vi "CleanUp.vi"(8 "error in (no error)":errorcluster, 11 "Prueba02 in":refnum<class "Prueba02.lvclass">) -> (0 "error out":errorcluster, 3 "Prueba02 out":refnum<class "Prueba02.lvclass">)   [LabVIEW 2019, in "Prueba02.lvclass"]
uses:
  Prueba02.lvclass
  C:/Users/ivan_/Documents/procal/Pruebas/Prueba/Prueba.lvclass
  Prueba/Prueba.lvclass/Prueba.ctl
  Prueba02.lvclass/Prueba02.ctl
  Base de Datos/SQLiteConnector/SQLiteConnection.lvclass
  Base de Datos/Base de Datos.lvclass
  Prueba/Prueba.lvclass
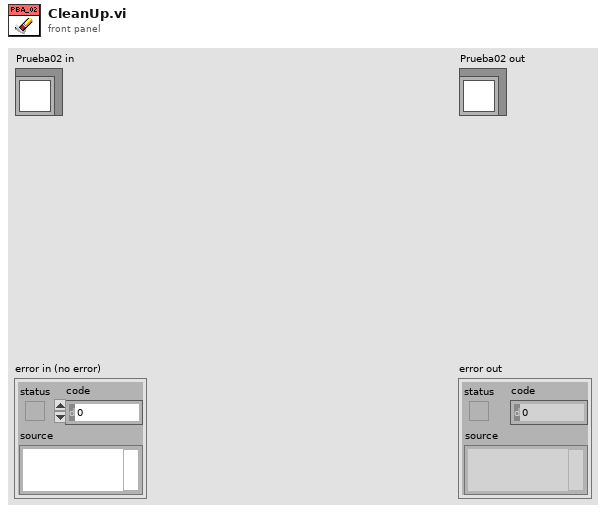
[diagram p1: front panel]
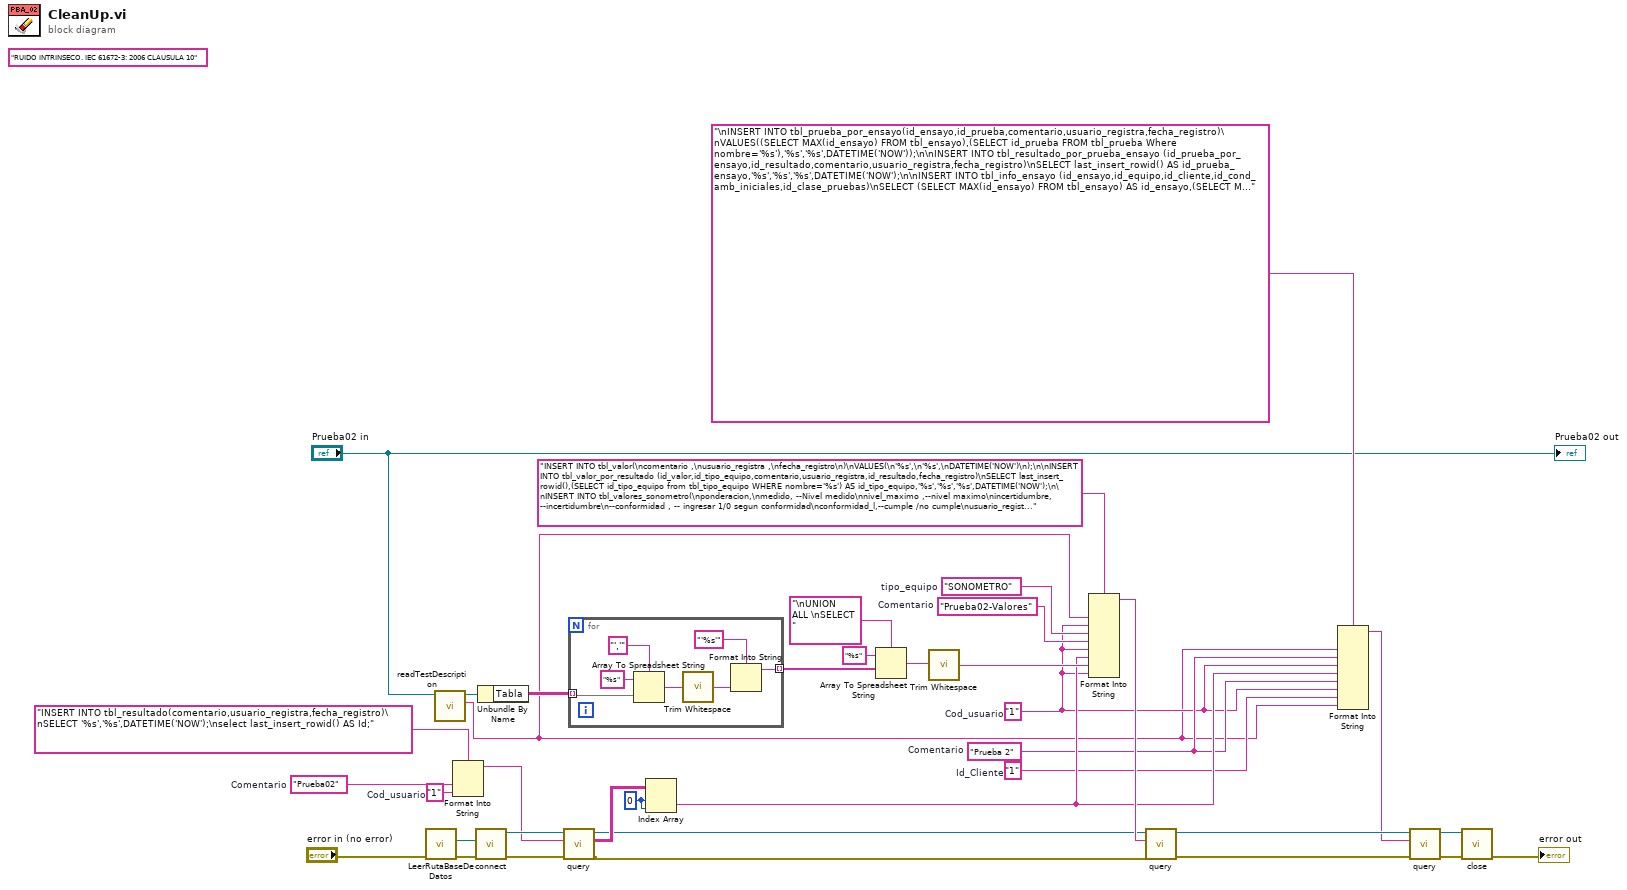
[diagram p0: block diagram]
diagram:
  (unwired) "RUIDO INTRINSECO. IEC 61672-3: 2006 CLAUSULA 10" ("input 2")
  w5 = "1"  # Id_Cliente
  w6 = "Prueba 2"  # Comentario
  w15 = "SONOMETRO"  # tipo_equipo
  w14 = "Prueba02-Valores"  # Comentario
  w21 = 0 ("index (row)")
  w23 = "1"  # Cod_usuario
  w24 = "Prueba02"  # Comentario
  w4 = "1"  # Cod_usuario
  n1 = call "LeerRutaBaseDeDatos.vi"("error in (no error)"="error in (no error)") -> ("error out"=w31:errorcluster, "Database Path"=w30:path)  [unwired: 9 in]
  n2 = call "readTestDescription.vi"("Prueba in"="Prueba02 in") -> ("Test Description"=w1:string, "Prueba out"=w2:refnum<class "Prueba02.lvclass">)  [unwired: 8 in, 1 out]
  n3 = Format Into String(format string="INSERT INTO tbl_resultado(comentario,usuario_registra,fecha_registro)\nSELECT '%s','%s',DATETIME('NOW');\nselect last_insert_rowid() AS Id;" ("SQL Statement"), w24, w23) -> (resulting string=w22:string)  [unwired: 2 in, 1 out]
  n4 = call "connect.vi"("error in (no error)"=w31, "Database Path"=w30) -> ("error out"=w20:errorcluster, "object out"=w26:refnum<class "SQLiteConnection.lvclass">)  [unwired: 8 in]
  n5 = Unbundle By Name(w2) -> ("Tabla"=w32:string[][])
  n6 = call "query.vi"("error in (no error)"=w20, "SQL Statement"=w22, "object in"=w26) -> ("error out"=w17:errorcluster, "result"=w19:string[][], "object out"=w18:refnum<class "SQLiteConnection.lvclass">)  [unwired: 5 in, 1 out]
  n7 = for {
    tunnel: w32 -> [w44] mode=indexing
    tunnel: [w40] -> w35 mode=indexing
    n8 = Array To Spreadsheet String(delimiter (Tab)="','", array=w44, 3:"%s" ("format string")) -> (spreadsheet string=w39:string)
    n9 = call <vilib>:"Trim Whitespace.vi"("string"=w39) -> ("trimmed string"=w38:string)  [unwired: 1 in]
    n10 = Format Into String(format string="'%s'", w38) -> (resulting string=w40:string)  [unwired: 2 in, 1 out]
  }
  n11 = Index Array(array=w19, index (row)=w21, index (col)=w21) -> (element=w7:string)
  n12 = Array To Spreadsheet String(delimiter (Tab)="\nUNION ALL \nSELECT ", array=w35, 3:"%s" ("format string")) -> (spreadsheet string=w34:string)
  n13 = call <vilib>:"Trim Whitespace.vi"("string"=w34) -> ("trimmed string"=w16:string)  [unwired: 1 in]
  n14 = Format Into String(format string="INSERT INTO tbl_valor(\ncomentario ,\nusuario_registra ,\nfecha_registro\n)\nVALUES(\n'%s',\n'%s',\nDATETIME('NOW')\n);\n\nINSERT INTO tbl_valor_por_resultado (id_valor,id_tipo_equipo,comentario,usuario_registra,id_resultado,fecha_registro)\nSELECT last_insert_rowid(),(SELECT id_tipo_equipo from tbl_tipo_equipo WHERE nombre='%s') AS id_tipo_equipo,'%s','%s','%s',DATETIME('NOW');\n\nINSERT INTO tbl_valores_sonometro(\nponderacion,\nmedido, --Nivel medido\nnivel_maximo ,--nivel maximo\nincertidumbre, --incertidumbre\n--conformidad , -- ingresar 1/0 segun conformidad\nconformidad_l,--cumple /no cumple\nusuario_registra,\nmedido_um , --(dB)\nnivel_maximo_um, --dB\nincertidumbre_um,--dB\n\nid_valor,\nfecha_registro\n)\nSELECT * FROM(\nSELECT %s\n) AS T\nINNER JOIN\n(SELECT %s AS usuario,'dB','dB','dB',(SELECT MAX(id_valor) FROM tbl_valor) AS id_valor,DATETIME('NOW') fecha ) AS F;\n", w1, w4, w15, w14, w4, w7, w16, w4) -> (resulting string=w27:string)  [unwired: 2 in, 1 out]
  n15 = call "query.vi"("error in (no error)"=w17, "SQL Statement"=w27, "object in"=w18) -> ("error out"=w11:errorcluster, "object out"=w13:refnum<class "SQLiteConnection.lvclass">)  [unwired: 5 in, 2 out]
  n16 = Format Into String(format string="\nINSERT INTO tbl_prueba_por_ensayo(id_ensayo,id_prueba,comentario,usuario_registra,fecha_registro)\nVALUES((SELECT MAX(id_ensayo) FROM tbl_ensayo),(SELECT id_prueba FROM tbl_prueba Where nombre='%s'),'%s','%s',DATETIME('NOW'));\n\nINSERT INTO tbl_resultado_por_prueba_ensayo (id_prueba_por_ensayo,id_resultado,comentario,usuario_registra,fecha_registro)\nSELECT last_insert_rowid() AS id_prueba_ensayo,'%s','%s','%s',DATETIME('NOW');\n\nINSERT INTO tbl_info_ensayo (id_ensayo,id_equipo,id_cliente,id_cond_amb_iniciales,id_clase_pruebas)\nSELECT (SELECT MAX(id_ensayo) FROM tbl_ensayo) AS id_ensayo,(SELECT MAX(id_equipo) FROM tbl_equipo) AS id_equipo,'%s' AS id_cliente,(SELECT MAX(id_cond_amb_iniciales) FROM tbl_cond_amb_iniciales) AS id_cond_amb_iniciales,\n(SELECT id_clase_prueba FROM tbl_clase_prueba WHERE id_clase=(SELECT id_clase FROM tbl_equipo ORDER BY id_equipo DESC LIMIT 1)  AND id_prueba=(SELECT id_prueba FROM tbl_prueba Where nombre='%s')) AS id_clase_pruebas;\n", w1, w6, w4, w7, w6, w4, w5, w1) -> (resulting string=w8:string)  [unwired: 2 in, 1 out]
  n17 = call "query.vi"("error in (no error)"=w11, "SQL Statement"=w8, "object in"=w13) -> ("error out"=w10:errorcluster, "object out"=w12:refnum<class "SQLiteConnection.lvclass">)  [unwired: 5 in, 2 out]
  n18 = call-dynamic "close.vi"("error in (no error)"=w10, "object in"=w12) -> ("error out"=→"error out":errorcluster)  [unwired: 8 in, 1 out]
  "Prueba02 out" <- "Prueba02 in"
